vi "Get Key Names.vi"(7 "Section Name":string, 8 "error in (no error)":errorcluster, 11 "Config in":refnum<class "LabVIEW-Config.lvclass">) -> (0 "error out":errorcluster, 1 "Key Names":string[](array[string]), 2 "Section Found?":bool, 3 "Config out":refnum<class "LabVIEW-Config.lvclass">)   [LabVIEW 2017, in "LabVIEW-Config.lvlib" / "LabVIEW-Config.lvclass"]
uses:
  LabVIEW-Config.lvclass
  LabVIEW-Config.lvclass/LabVIEW-Config.ctl
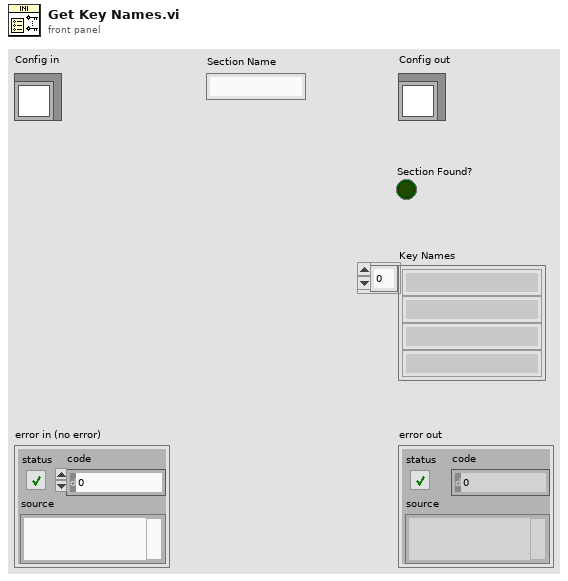
[diagram p1: front panel]
types:
  T1 = typedef "LabVIEW-Config.lvlib/LabVIEW-Config.lvclass/LineToken.ctl" = enum8{"comment", "section", "key", "more"}
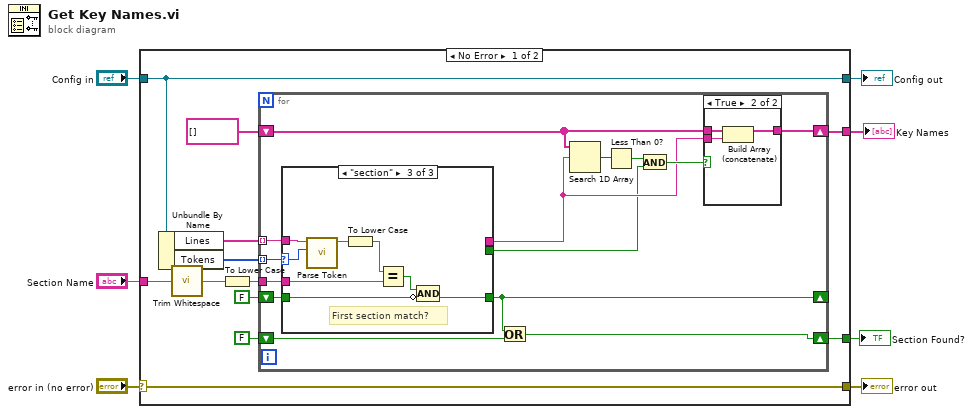
[diagram p0: block diagram]
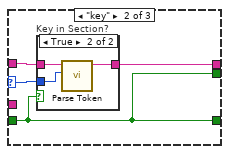
[diagram p4: hidden frame]
diagram:
  n1 = case shown="No Error" "error in (no error)" {
    selector: "error in (no error)" -> [w18 w55]
    tunnel: "Config in" -> [w17 w54]
    tunnel: [w9 _] -> w6
    tunnel: [w18 w55] -> w5
    tunnel: [w17 w54] -> w3
    tunnel: "Section Name" -> [w16 _]
    tunnel: [w12 _] -> w1
    frame No Error {
      n2 = Unbundle By Name(w17) -> ("Lines"=w19:string[], "Tokens"=w11:T1[])
      n3 = call <vilib>:"Trim Whitespace.vi"("string"=w16) -> ("trimmed string"=w8:string)  [unwired: 1 in]
      n4 = To Lower Case(string=w8) -> (all lower case string=w15:string)
      n5 = for {
        tunnel: w11 -> [w33] mode=indexing
        tunnel: w19 -> [w32] mode=indexing
        tunnel: w15 -> [w31]
        shift-right: [w29] -> _
        shift-left: FALSE -> [w30]
        shift-right: [w28] -> w12
        shift-left: FALSE -> [w27]
        shift-right: [w23] -> w9
        shift-left: string[] [] -> [w22]
        n6 = case shown="\"section\"" w33 {
          selector: w33 -> [_ w39 w46]
          tunnel: w32 -> [_ w42 w48]
          tunnel: [_ w41 _] -> w21
          tunnel: w31 -> [_ _ w53]
          tunnel: [w38 w40 w49] -> w29
          tunnel: w30 -> [w38 w40 w51]
          tunnel: [_ w40 _] -> w20
          frame "comment", "more" {
          }
          frame "key" {
            n7 = case "Key in Section?" shown="True" w40 {
              tunnel: w42 -> [_ w45]
              tunnel: [_ w43] -> w41
              tunnel: w39 -> [_ w44]
              frame False {
              }
              frame True {
                n8 = call "Parse Token.vi"("Token"=w44, "Line"=w45) -> ("Name"=w43:string)  [unwired: 8 in, 1 out]
              }
            }
          }
          frame "section" {
            # "First section match?"
            n9 = call "Parse Token.vi"("Token"=w46, "Line"=w48) -> ("Name"=w47:string)  [unwired: 8 in, 1 out]
            n10 = To Lower Case(string=w47) -> (all lower case string=w52:string)
            n11 = Equal?(x=w52, y=w53) -> (x = y?=w50:bool)
            n12 = Compound Arithmetic op=AND(w50, invert w51) -> (w49:bool)
          }
        }
        n13 = Or(x=w29, y=w27) -> (x .or. y?=w28:bool)
        n14 = Search 1D Array(1D array=w22, element=w21) -> (index of element=w26:i32)  [unwired: 1 in]
        n15 = Less Than 0?(x=w26) -> (x < 0?=w25:bool)
        n16 = And(x=w25, y=w20) -> (x .and. y?=w24:bool)
        n17 = case shown="True" w24 {
          tunnel: [w34 w37] -> w23
          tunnel: w22 -> [w34 w36]
          tunnel: w21 -> [_ w35]
          frame False {
          }
          frame True {
            n18 = Build Array (concatenate)(w36, w35) -> (w37:string[])
          }
        }
      }
    }
    frame Error {
    }
  }
  "error out" <- w5
  "Config out" <- w3
  "Key Names" <- w6
  "Section Found?" <- w1
